vi "TEMP STAB.vi"(0 "Queue in":refnum<queue>, 1 "element in":T1 {"Output's Control Loop (1:1)" items=["1"=1, "2"=2]; "Data Source (0:Kelvin)" items=["Kelvin", "Celsius", "Sensor Units"]; "Input (0:A)" items=["A", "B", "C", "D", "D2", "D3", "D4", "D5"]; "Configure Control Parameters (0: Configure)" items=["Configure", "Don't Configure"]; "Serial Configuration"."Flow Control" items=["None", "XON/XOFF", "RTS/CTS", "XON/XOFF & RTS/CTS", "DTR/DSR", "XON/XOFF & DTR/DSR"]; "Serial Configuration"."Stop Bits" items=["1.0"=10, "1.5"=15, "2.0"=20]; "Serial Configuration"."Data Bits" items=["7"=7, "8"=8]; "Serial Configuration"."Parity" items=["None", "Odd", "Even", "Mark", "Space"]; "Serial Configuration"."Baud Rate" items=["300"=300, "600"=600, "1200"=1200, "2400"=2400, "4800"=4800, "9600"=9600, "19200"=19200, "38400"=38400, "57600"=57600]; "Target Temp (K)" format="%.5f"; "Input (0:None)" items=["None", "A", "B", "C", "D", "D2", "D3", "D4", "D5"]; "Mode (0:Off)" items=["Off", "Closed Loop PID", "Zone", "Open Loop"]; "Heater Out Display (1:Current)" items=["Current"=1, "Power"=2]; "Max Current (0:User Specified)" items=["User Specified", "0.707 A", "1.0 A", "1.141 A", "2.0 A"]; "Heater Resistance (1:25 Ohms)" items=["25 Ohms"=1, "50 Ohms"=2]; "Max User Current (2.000)" format="%.3f"; "Gain (P) (50.0)" format="%.1f"; "Reset (I) (20.0)" format="%.1f"; "Rate (D) (0.0 %)" format="%.1f"; "Manual Output (0.00 %)" format="%.2f"; "Range (0:Off)" items=["Off", "Range 1 (On)", "Range 2", "Range 3", "Range 4", "Range 5"]}, 5 "element 2":dbl[](array[numeric]), 7 "ScanQ In":refnum<queue>, 9 "Setpoint":dbl, 11 "error in (no error)":errorcluster, 12 "element":dbl) -> (4 "Queue out":refnum<queue>, 6 "Array out":dbl[](array[numeric]), 8 "ScanQ":refnum<queue>, 10 "element out":T1 {"Output's Control Loop (1:1)" items=["1"=1, "2"=2]; "Data Source (0:Kelvin)" items=["Kelvin", "Celsius", "Sensor Units"]; "Input (0:A)" items=["A", "B", "C", "D", "D2", "D3", "D4", "D5"]; "Configure Control Parameters (0: Configure)" items=["Configure", "Don't Configure"]; "Serial Configuration"."Flow Control" items=["None", "XON/XOFF", "RTS/CTS", "XON/XOFF & RTS/CTS", "DTR/DSR", "XON/XOFF & DTR/DSR"]; "Serial Configuration"."Stop Bits" items=["1.0"=10, "1.5"=15, "2.0"=20]; "Serial Configuration"."Data Bits" items=["7"=7, "8"=8]; "Serial Configuration"."Parity" items=["None", "Odd", "Even", "Mark", "Space"]; "Serial Configuration"."Baud Rate" items=["300"=300, "600"=600, "1200"=1200, "2400"=2400, "4800"=4800, "9600"=9600, "19200"=19200, "38400"=38400, "57600"=57600]; "Target Temp (K)" format="%.5f"; "Input (0:None)" items=["None", "A", "B", "C", "D", "D2", "D3", "D4", "D5"]; "Mode (0:Off)" items=["Off", "Closed Loop PID", "Zone", "Open Loop"]; "Heater Out Display (1:Current)" items=["Current"=1, "Power"=2]; "Max Current (0:User Specified)" items=["User Specified", "0.707 A", "1.0 A", "1.141 A", "2.0 A"]; "Heater Resistance (1:25 Ohms)" items=["25 Ohms"=1, "50 Ohms"=2]; "Max User Current (2.000)" format="%.3f"; "Gain (P) (50.0)" format="%.1f"; "Reset (I) (20.0)" format="%.1f"; "Rate (D) (0.0 %)" format="%.1f"; "Manual Output (0.00 %)" format="%.2f"; "Range (0:Off)" items=["Off", "Range 1 (On)", "Range 2", "Range 3", "Range 4", "Range 5"]}, 15 "error out":errorcluster)   [LabVIEW 2025]
uses:
  <vilib>/Analysis/NI_AALBase.lvlib
  <vilib>/Analysis/baseanly.llb/Mean (DBL).vi
  Labview-File/STM-Auto-Project Testing/STM-Auto-Project (Trial 2)/QMH CTLS/Scan_Params (QMH).ctl
  <userlib>/Nanonis Prog Interface V5e/Nanonis Prog Interface.lvlib
  Temp Cntrl.ctl
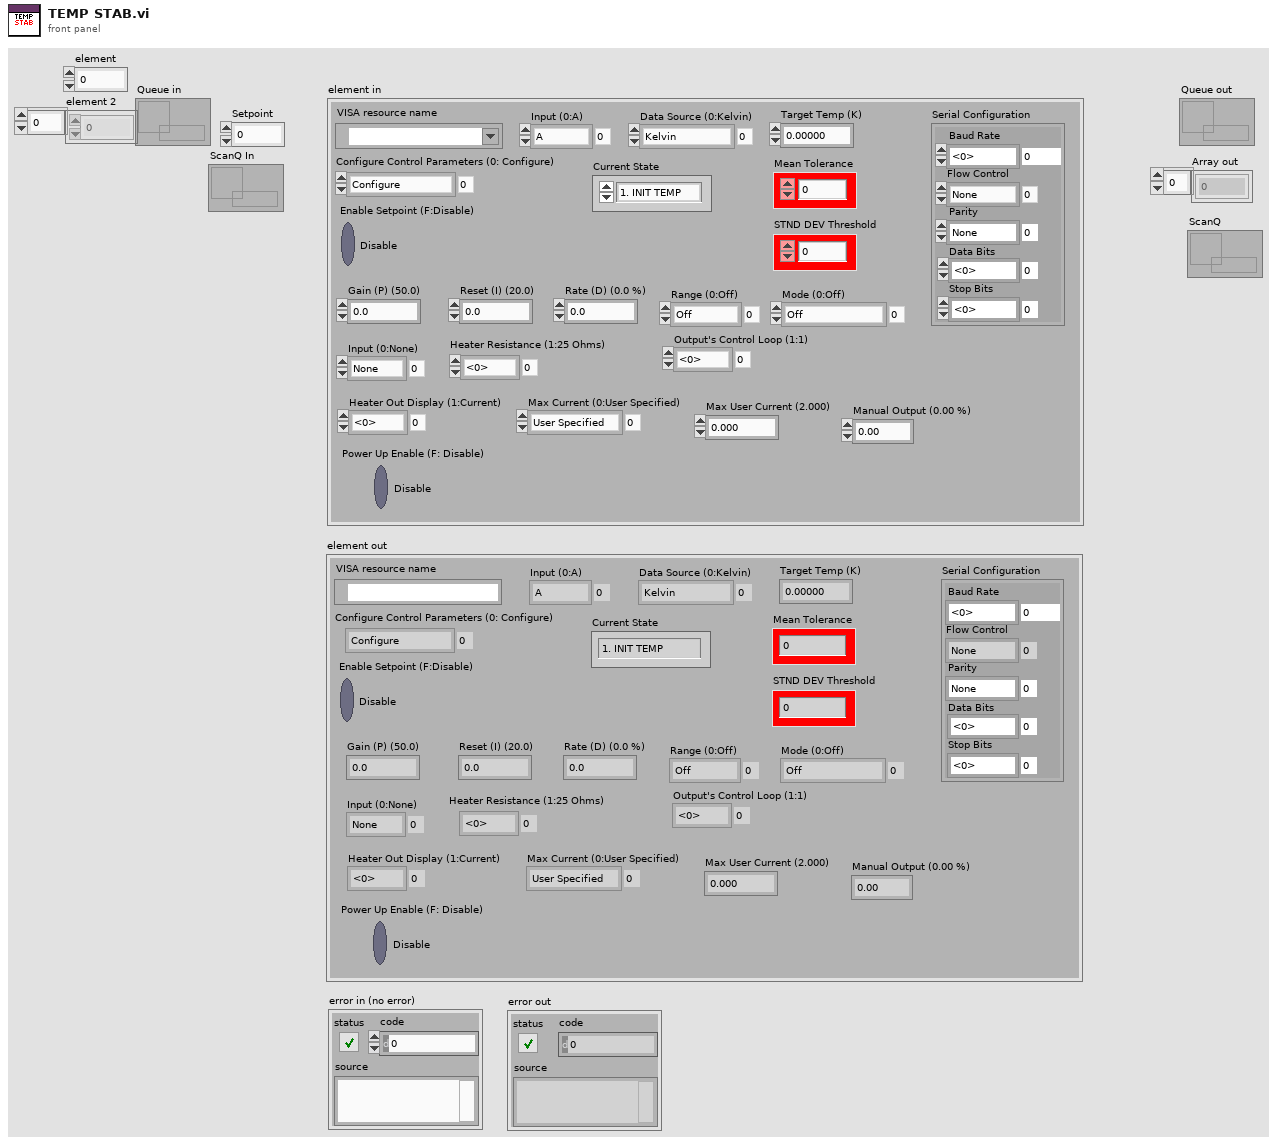
[diagram p1: front panel]
types:
  T1 = typedef "Temp Cntrl.ctl" = cluster{"Range (0:Off)":u16, "Manual Output (0.00 %)":dbl, "Rate (D) (0.0 %)":dbl, "Reset (I) (20.0)":dbl, "Gain (P) (50.0)":dbl, "Power Up Enable (F: Disable)":bool, "Max User Current (2.000)":dbl, "Heater Resistance (1:25 Ohms)":u16, "Max Current (0:User Specified)":u16, "Heater Out Display (1:Current)":u16, "Mode (0:Off)":u16, "Input (0:None)":u16, "Target Temp (K)":dbl, "Serial Configuration":cluster{"Baud Rate":u32, "Parity":u16, "Data Bits":u16, "Stop Bits":u16, "Flow Control":u16}, "VISA resource name":refnum<visa-resource-name>, "Configure Control Parameters (0: Configure)":u16, "Enable Setpoint (F:Disable)":bool, "Input (0:A)":u16, "Data Source (0:Kelvin)":u16, "Output's Control Loop (1:1)":u16, "STND DEV Threshold ":dbl, "Mean Tolerance ":dbl, "Current State":enum16{"1. INIT TEMP", "2. TC ON", "3. POLL_TEMPS", "4. TEMP_STAB", "5. TC IDLE", "6. APPLY NEXT TEMP", "7. TC OFF (Reset)"}}
  T2 = enum16{"1. INIT TEMP", "2. TC ON", "3. POLL_TEMPS", "4. TEMP_STAB", "5. TC IDLE", "6. APPLY NEXT TEMP", "7. TC OFF (Reset)"}
  T3 = enum16{"1. BIAS", "2. INIT_SCAN", "3. SCAN_IDLE", "4. INTER_SCAN", "5. NEW_COORDS_&_FRAME", "6. FINAL_SCAN", "7. POLL_BIAS", "8. Z-CONT.", "9. STOP"}
  T4 = typedef "Scan_Params (QMH).ctl" = cluster{"Setpoint (I)":dbl[], "Bias (V)":dbl[], "Number of scans":u8, "Port number (3364)":u32, "Avoid zero threshold (V)":dbl, "Current State":enum16{"1. BIAS", "2. INIT_SCAN", "3. SCAN_IDLE", "4. INTER_SCAN", "5. NEW_COORDS_&_FRAME", "6. FINAL_SCAN", "7. STOP"}}
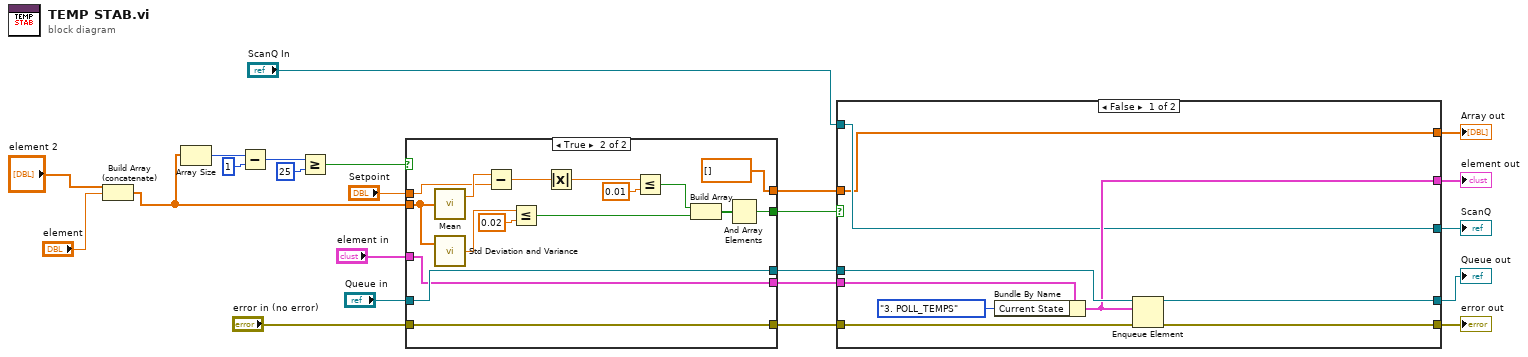
[diagram p0: block diagram]
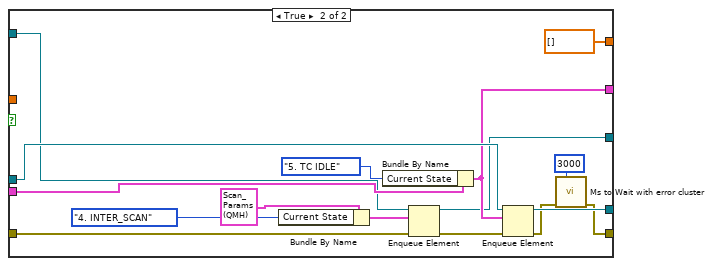
[diagram p2: hidden frame]
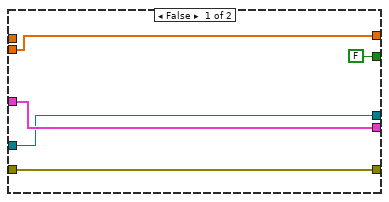
[diagram p3: hidden frame]
diagram:
  n1 = Build Array (concatenate)("element 2", "element") -> (w6:dbl[])
  n2 = Array Size(array=w6) -> (size(s)=w9:i32)
  n3 = Subtract(x=w9, y=1) -> (x-y=w11:i32)
  n4 = Greater Or Equal?(x=w11, y=25) -> (x >= y?=w4:bool)
  n5 = case shown="True" w4 {
    tunnel: "Setpoint" -> [_ w40]
    tunnel: w6 -> [w24 w29]
    tunnel: [FALSE w34] -> w16
    tunnel: "Queue in" -> [w27 w33]
    tunnel: "element in" -> [w28 w32]
    tunnel: "error in (no error)" -> [w26 w31]
    tunnel: [w27 w33] -> w17
    tunnel: [w26 w31] -> w18
    tunnel: [w28 w32] -> w19
    tunnel: [w24 dbl[] []] -> w5
    frame False {
    }
    frame True {
      n6 = call-poly <vilib>:"Mean.vi"("X"=w29) -> ("mean"=w42:dbl)  [unwired: 1 out]
      n7 = call <vilib>:"Std Deviation and Variance.vi"("X"=w29) -> ("standard deviation"=w44:dbl)  [unwired: 1 in, 2 out]
      n8 = Subtract(x=w42, y=w40) -> (x-y=w41:dbl)
      n9 = Less Or Equal?(x=w44, y=0.02) -> (x <= y?=w36:bool)
      n10 = Absolute Value(x=w41) -> (abs(x)=w39:dbl)
      n11 = Less Or Equal?(x=w39, y=0.01) -> (x <= y?=w37:bool)
      n12 = Build Array(w37, w36) -> (w35:bool[])
      n13 = And Array Elements(Boolean array=w35) -> (logical AND=w34:bool)
    }
  }
  n14 = case shown="False" w16 {
    tunnel: w17 -> [w53 w69]
    tunnel: w18 -> [w49 w61]
    tunnel: w19 -> [w52 w68]
    tunnel: [w51 w67] -> w20
    tunnel: [w50 w54] -> w21
    tunnel: [w45 dbl[] []] -> w1
    tunnel: [w48 w66] -> w23
    tunnel: "ScanQ In" -> [w47 w65]
    tunnel: [w47 w62] -> w8
    tunnel: w5 -> [w45 _]
    frame False {
      n15 = Bundle By Name(cluster=w52, "Current State"=T2."3. POLL_TEMPS") -> (w48:T1)
      n16 = Enqueue Element(queue=w53, element=w48, error in (no error)=w49) -> (queue out=w51:refnum<queue>, error out=w50:errorcluster)  [unwired: 1 in, 1 out]
    }
    frame True {
      n17 = Bundle By Name(cluster=T4 {"Setpoint (I)"=[], "Bias (V)"=[], "Number of scans"=1, "Port number (3364)"=3364, "Avoid zero threshold (V)"=0.004999999888241291, "Current State"=enum."1. BIAS"} ("element"), "Current State"=T3."4. INTER_SCAN") -> (w63:T4)
      n18 = Bundle By Name(cluster=w68, "Current State"=T2."5. TC IDLE") -> (w66:T1)
      n19 = Enqueue Element(queue=w65, element=w63, error in (no error)=w61) -> (queue out=w62:refnum<queue>, error out=w60:errorcluster)  [unwired: 1 in, 1 out]
      n20 = Enqueue Element(queue=w69, element=w66, error in (no error)=w60) -> (queue out=w67:refnum<queue>, error out=w55:errorcluster)  [unwired: 1 in, 1 out]
      n21 = call <userlib>:"Ms to Wait with error cluster.vi"("error in (no error)"=w55, "milliseconds to wait"=u32 3000) -> ("error out"=w54:errorcluster)  [unwired: 4 in, 1 out]
    }
  }
  "element out" <- w23
  "Array out" <- w1
  "error out" <- w21
  "Queue out" <- w20
  "ScanQ" <- w8
